vi "Funktionsgenerator - Kopie.vi"() -> ()   [LabVIEW 2017]
uses:
  <vilib>/Utility/error.llb/DialogType.ctl
  <vilib>/DAQmx/read.llb/DAQmx Read (Analog Wfm 1Chan NSamp).vi
  <vilib>/DAQmx/create/channels.llb/DAQmx Create Channel (AI-Voltage-Basic).vi
  <vilib>/DAQmx/configure/timing.llb/DAQmx Timing (Sample Clock).vi
  <vilib>/DAQmx/miscellaneous.llb/DAQmx Fill In Error Info.vi
  <vilib>/express/express analysis/Spectral/Block/exnSpectralBlock spectral measurements power poly.vi
  <vilib>/express/express analysis/Spectral/Block/exnSpectralBlock spectral measurements power WFM.vi
  <vilib>/express/express analysis/Spectral/XNode/ExpressSpectralMeasurementsBlockNode.xnode
panel:
  out "Waveform Graph 2":cluster{"f0":dbl, "df":dbl, "magnitude":dbl[]}(graph)
  in  "stop":bool
  out "Waveform Graph":waveform(dbl)(graph)
  in  "minimum value":dbl=-5.0 format="%0.2f"
  in  "maximum value":dbl=5.0 format="%0.2f"
  in  "rate":dbl=1000.0 format="%0.2f"
  in  "physical channels":tag
  in  "samples per channel":i32=1000
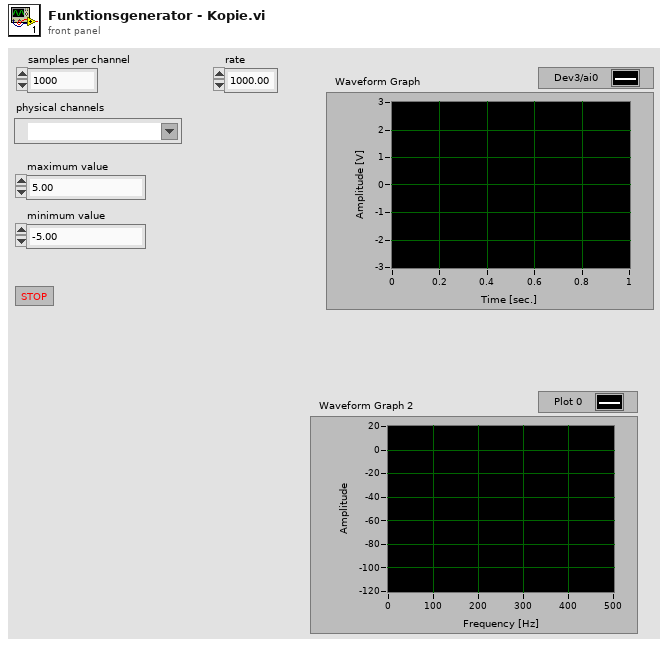
[diagram p1: front panel]
types:
  T1 = cluster{"averaging mode":u16, "weighting mode":u16, "number of averages":u32}
  T2 = cluster{"dB On (F)":bool, "unwrap phase (F)":bool, "convert to degree (F)":bool}
  T3 = typedef "DialogType.ctl" = u16
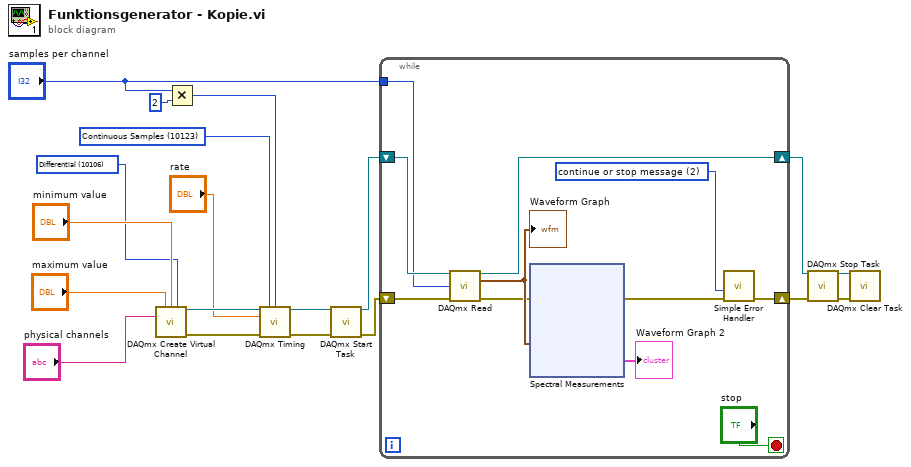
[diagram p0: block diagram]
diagram:
  w5 = 10123 items=["Finite Samples"=10178, "Continuous Samples"=10123, "Hardware Timed Single Point"=12522] ("sample mode")
  w3 = 10106 items=["Default"=-1, "RSE"=10083, "NRSE"=10078, "Differential"=10106, "Pseudodifferential"=12529] ("input terminal configuration")
  n1 = call-poly <vilib>:"DAQmx Create Virtual Channel.vi"("maximum value"="maximum value", "minimum value"="minimum value", "input terminal configuration"=w3, "physical channels"="physical channels") -> ("task out"=w14:refnum<k21>, "error out"=w19:errorcluster)  [unwired: 10 in]
  n2 = Multiply(x="samples per channel", y=2 ("x*y")) -> (x*y=w2:i32)
  n3 = call-poly <vilib>:"DAQmx Timing.vi"("task/channels in"=w14, "sample mode"=w5, "samples per channel"=w2, "rate"="rate", "error in"=w19) -> ("task out"=w13:refnum<k21>, "error out"=w18:errorcluster)  [unwired: 9 in]
  n4 = call <vilib>:"DAQmx Start Task.vi"("task/channels in"=w13, "error in"=w18) -> ("task out"=w12:refnum<k21>, "error out"=w17:errorcluster)  [unwired: 12 in]
  n5 = while {
    shift-right: [w25] -> w16
    shift-left: w17 -> [w30]
    shift-right: [w28] -> w11
    shift-left: w12 -> [w29]
    tunnel: "samples per channel" -> [w26]
    stop <- "stop" stop-if-true
    w24 = T3 2 items=["no dialog", "OK message", "continue or stop message", "OK message + warnings", "continue/stop + warnings"] ("type of dialog (OK msg:1)")
    n6 = call-poly <vilib>:"DAQmx Read.vi"("task/channels in"=w29, "number of samples per channel"=w26, "error in"=w30) -> ("task out"=w28:refnum<k21>, "data"=w23:waveform(dbl), "error out"=w22:errorcluster)  [unwired: 10 in]
    "Waveform Graph" <- w23
    n7 = xnode "Spectral Measurements"("Signals"=w23, "error in (no error)"=w22) -> ("Power Spectrum"=→"Waveform Graph 2":cluster{"f0":dbl, "df":dbl, "magnitude":dbl[]}, "error out"=w20:errorcluster)
    n8 = call <vilib>:"Simple Error Handler.vi"("type of dialog (OK msg:1)"=w24, "error in (no error)"=w20) -> ("error out"=w25:errorcluster)  [unwired: 3 in, 4 out]
  }
  n9 = call <vilib>:"DAQmx Stop Task.vi"("task/channels in"=w11, "error in"=w16) -> ("task out"=w10:refnum<k21>, "error out"=w15:errorcluster)  [unwired: 12 in]
  n10 = call <vilib>:"DAQmx Clear Task.vi"("task in"=w10, "error in"=w15) -> ()  [unwired: 13 in, 1 out]
